vi "Convert filetype to Can be in LLB.vi"(4 "file type":T1) -> (1 "Can be in LLB?":bool)   [LabVIEW 2018, in "NI_FileType.lvlib"]
doc: "Returns TRUE if this file type could be copied into an LLB."
uses:
  NI_FileType.lvlib
  FT_FileTypes.ctl
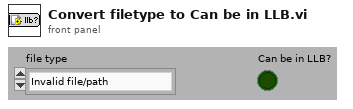
[diagram p1: front panel]
types:
  T1 = typedef "NI_FileType.lvlib/FT_FileTypes.ctl" = enum32{"Invalid file/path", "Unknown type", "Instrument", "Control", "Polymorphic VI", "Project", "Library", "LVClass", "XControl", "XNode", "CIN", "Run-time menu", "Palette menu", "LLB", "Shortcut", "Directory", "Class Private Data Control", "Statechart", "MathScript .m file", "Ladder Diagram", "LVLibp"}
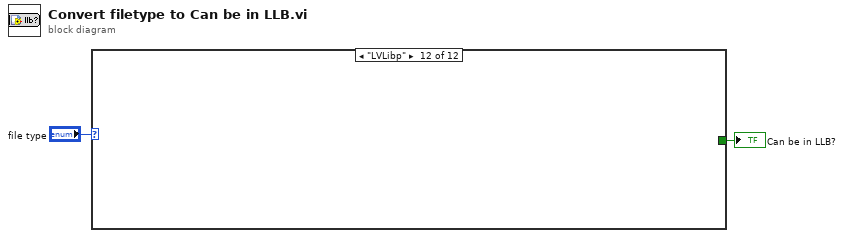
[diagram p0: block diagram]
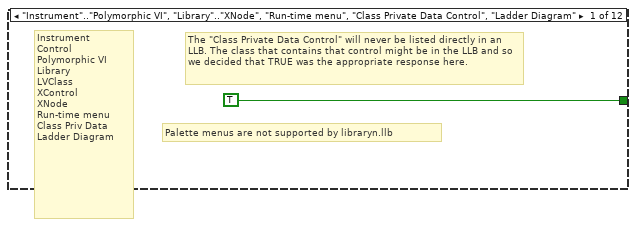
[diagram p2: hidden frame]
diagram:
  n1 = case shown="\"LVLibp\"" "file type" {
    tunnel: [TRUE _ _ _ _ _ _ _ _ _ _ _] -> w1
    frame "Instrument".."Polymorphic VI", "Library".."XNode", "Run-time menu", "Class Private Data Control", "Ladder Diagram" {
      # "The \"Class Private Data Control\" will never be listed directly in an LLB. The class that contains that control might be in the LLB and so we decided that TRUE was the appropriate response here."
      # "Palette menus are not supported by libraryn.llb"
      # "Instrument\nControl\nPolymorphic VI\nLibrary\nLVClass\nXControl\nXNode\nRun-time menu\nClass Priv Data\nLadder Diagram"
    }
    frame "Project" {
    }
    frame "CIN" {
    }
    frame "Palette menu" {
    }
    frame "LLB" {
    }
    frame "Shortcut" {
    }
    frame "Directory" {
    }
    frame "Unknown type" {
    }
    frame "Invalid file/path" {
    }
    frame "Statechart" {
    }
    frame "MathScript .m file" {
    }
    frame "LVLibp" {
    }
  }
  "Can be in LLB?" <- w1
